vi "軟體極限.vi"(11 "Boolean":bool) -> (3 "Disabled":T1(ring))   [LabVIEW 2015]
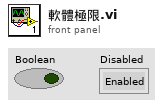
[diagram p1: front panel]
types:
  T1 = enum8{"Enabled", "Disabled", "Disabled and Grayed Out"}
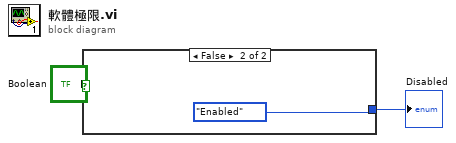
[diagram p0: block diagram]
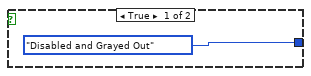
[diagram p2: hidden frame]
diagram:
  n1 = case shown="False" "Boolean" {
    tunnel: [T1."Disabled and Grayed Out" ("Disabled") T1."Enabled" ("Disabled")] -> w2
    frame True {
    }
    frame False {
    }
  }
  "Disabled" <- w2
